vi "Read RM Addresses.vi"(6 "FIFO Idxs":i32[](array[numeric]), 8 "error in":errorcluster, 9 "Session":refnum<visa-resource-name>, 10 "Addresses":u32[](array[numeric]), 11 "Old Values":dbl[](array[numeric])) -> (0 "error out":errorcluster, 2 "Read Duration":u32, 3 "Updated Values":dbl[](array[numeric]))   [LabVIEW 2010, in "RefMem PtByPt Custom Device.lvlib"]
uses:
  RefMem PtByPt Custom Device.lvlib
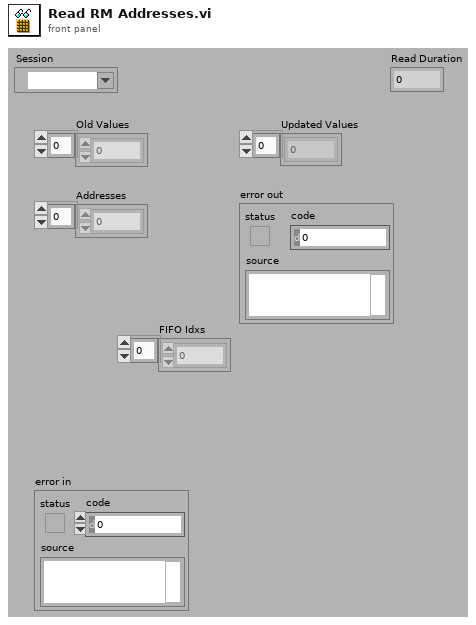
[diagram p1: front panel]
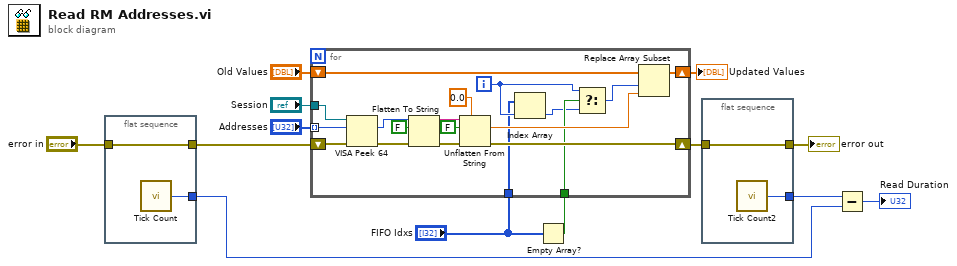
[diagram p0: block diagram]
diagram:
  n1 = flat-sequence {
    tunnel: [w15] -> w10
    tunnel: "error in" -> [w15]
    tunnel: [w14] -> w5
    frame #0 {
      n2 = call "Tick Count"() -> ("Tick Count(uSec)"=w14:u32)
    }
  }
  n3 = Empty Array?(array="FIFO Idxs") -> (empty?=w2:bool)
  n4 = for "Write Output Values to System" {
    shift-right: [w29] -> w8
    shift-left: w10 -> [w32]
    shift-right: [w33] -> w11
    shift-left: "Old Values" -> [w34]
    tunnel: "Addresses" -> [w26] mode=indexing
    tunnel: "Session" -> [w25]
    tunnel: w2 -> [w23]
    tunnel: "FIFO Idxs" -> [w21]
    i -> [w22]
    n5 = VISA Peek 64(8:w32, 10:w26, 11:w25) -> (0:w30:errorcluster, 2:w28:u64)  [unwired: 1 out]
    n6 = Flatten To String(anything=w28, prepend array or string size? (T)=FALSE, error in (no error)=w30) -> (data string=w18:string, error out=w17:errorcluster)  [unwired: 1 in, 1 out]
    n7 = Unflatten From String(type=0.0, binary string=w18, data includes array or string size? (T)=FALSE, error in (no error)=w17) -> (value=w27:dbl, error out=w29:errorcluster)  [unwired: 1 in, 1 out]
    n8 = Index Array(array=w21, index=w22) -> (element=w20:i32)
    n9 = Select(t=w22, s=w23, f=w20) -> (s? t:f=w24:i32)
    n10 = Replace Array Subset(array=w34, new element=w27, index=w24) -> (w33:dbl[])
  }
  "Updated Values" <- w11
  n11 = flat-sequence {
    tunnel: [w36] -> w7
    tunnel: w8 -> [w36]
    tunnel: [w35] -> w6
    frame #0 {
      n12 = call "Tick Count2"() -> ("Tick Count(uSec)"=w35:u32)
    }
  }
  n13 = Subtract(x=w6, y=w5) -> (x-y=→"Read Duration":u32)
  "error out" <- w7
